vi "AlazarBoardsFound.vi"(0 "error in (no error)":errorcluster) -> (1 "Boards Found":u32, 2 "error out":errorcluster)   [LabVIEW 2009]
doc: "Determine the number of digitizer boards that were detected in all board systems."
uses:
  ATSApi.dll
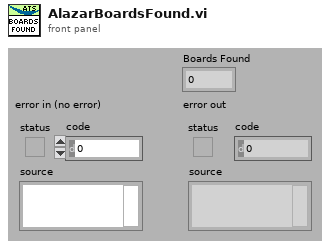
[diagram p1: front panel]
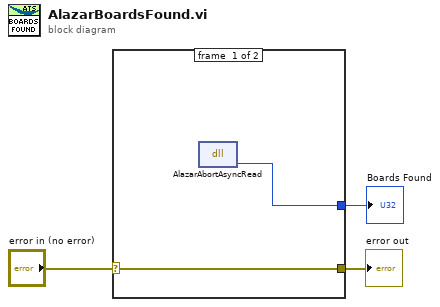
[diagram p0: block diagram]
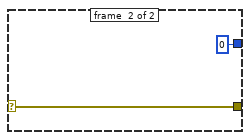
[diagram p2: hidden frame]
diagram:
  n1 = case shown="No Error" "error in (no error)" {
    selector: "error in (no error)" -> [w4 w7]
    tunnel: [w4 w7] -> w2
    tunnel: [w5 u32 0] -> w1
    frame #0 {
      n2 = dll-call lib="ATSApi.dll" fn="AlazarAbortAsyncRead"() -> (w5:u32)  [unwired: 3 in, 2 out]
    }
    frame #1 {
    }
  }
  "error out" <- w2
  "Boards Found" <- w1
